vi "CST_RegMap Item.vi"() -> (0 "RegMap Item":T1 {"Mask" format="%.0x"})   [LabVIEW 2010]
uses:
  TYP_RegMap Item.ctl
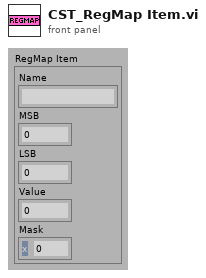
[diagram p1: front panel]
types:
  T1 = typedef "TYP_RegMap Item.ctl" = cluster{"Name":string, "MSB":u16, "LSB":u16, "Value":u16, "Mask":u16}
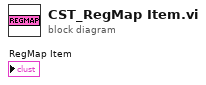
[diagram p0: block diagram]
diagram:
